vi "CANopen Read CAN Frame.vi"() -> ()   [LabVIEW 2016]
doc: "This example demonstrates how to read a raw CAN frame from CAN bus."
uses:
  <vilib>/userdefined/High Color/nirio_resource_hc.ctl
  <vilib>/Platform/TimedLoop/XDataNode/timing_clust.ctl
  <vilib>/Platform/TimedLoop/XDataNode/nitl_modes.ctl
  <vilib>/Platform/TimedLoop/XDataNode/wakeup.ctl
  <vilib>/FPGAPlugInAG/cRIO-9033/niLvFpga_Open_cRIO-9033.vi
  <vilib>/rvi/interface/common/dynamic/niFpgaDynamicAddResources.vi
  <vilib>/CANopenLib/CANOPEN.llb/CANopen Interface Create.vi
  <vilib>/CANopenLib/CANOPEN.llb/CANopen CAN Frame Read Create.vi
  <vilib>/CANopenLib/CANOPEN.llb/CANopen CAN Frame Read Start.vi
  <vilib>/CANopenLib/CANOPEN.llb/CANopen CAN Frame Read Close.vi
  <vilib>/CANopenLib/CANOPEN.llb/CANopen Interface Close.vi
  <vilib>/FPGAPlugInAG/Dynamic/niLvFpga_Close_Dynamic.vi
  <vilib>/rvi/interface/nirviOpenFPGA/nirviOpenFPGA.xnode
  FPGA Bitfiles/project_FPGATarget_MainFPGA_S9ZLErdeBuw.lvbitx
  FPGA/MainFPGA.vi
  <vilib>/Platform/TimedLoop/XDataNode/XDataNode.xnode
  <vilib>/rvi/interface/nirviCloseFPGA/nirviCloseFPGA.xnode
  <vilib>/Platform/TimedLoop/XDataNode/XDNodeRunTimeDep.lvlib
panel:
  in  "error in":errorcluster
  out "CAN message data":u8[](array[numeric])
  in  "period (ms)":i64=10
  out "COB-ID":u32 format="%.0x"
  out "RTR?":bool
  out "timestamp":timestamp
  out "New Data?":bool
  in  "stop":bool
  in  "buffer size (0)":u16=5
  in  "node-ID":u8=1 min=1 max=127 step=1
  in  "baud rate":u32(ring)=2 items=["1 Mbit/s"=0, "800 kbit/s"=1, "500 kbit/s"=2, "250 kbit/s"=3, "125 kbit/s"=4, "50 kbit/s"=6, "20 kbit/s"=7, "10 kbit/s"=8]
  in  "CANopen interface":u32(ring) items=["CANopen01", "CANopen02", "CANopen03", "CANopen04", "CANopen05", "CANopen06", "CANopen07", "CANopen08", "CANopen09", "CANopen10", "CANopen11", "CANopen12", "CANopen13", "CANopen14", "CANopen15", "CANopen16", "CANopen17", "CANopen18", "CANopen19", "CANopen20", "CANopen21", "CANopen22", "CANopen23", "CANopen24", "CANopen25", "CANopen26", "CANopen27", "CANopen28", "CANopen29", "CANopen30", "CANopen31", "CANopen32"]
  # "Overview: This example demonstrates how to read a raw CAN frame from CAN bus.  \nRequirements: Connect CANopen module with a slave device.\nInstructions:\n1. Specify the values of CANopen interface, baud rate of the CANopen interface, node-ID of the slave device and\n    buffer size (0) of the maximum number of CAN frames that the buffer saves.\n2. Run the VI.\n3. Click STOP to stop the VI."
  # "Create CANopen interface and raw CAN Frame object"
  # "Read CAN messages"
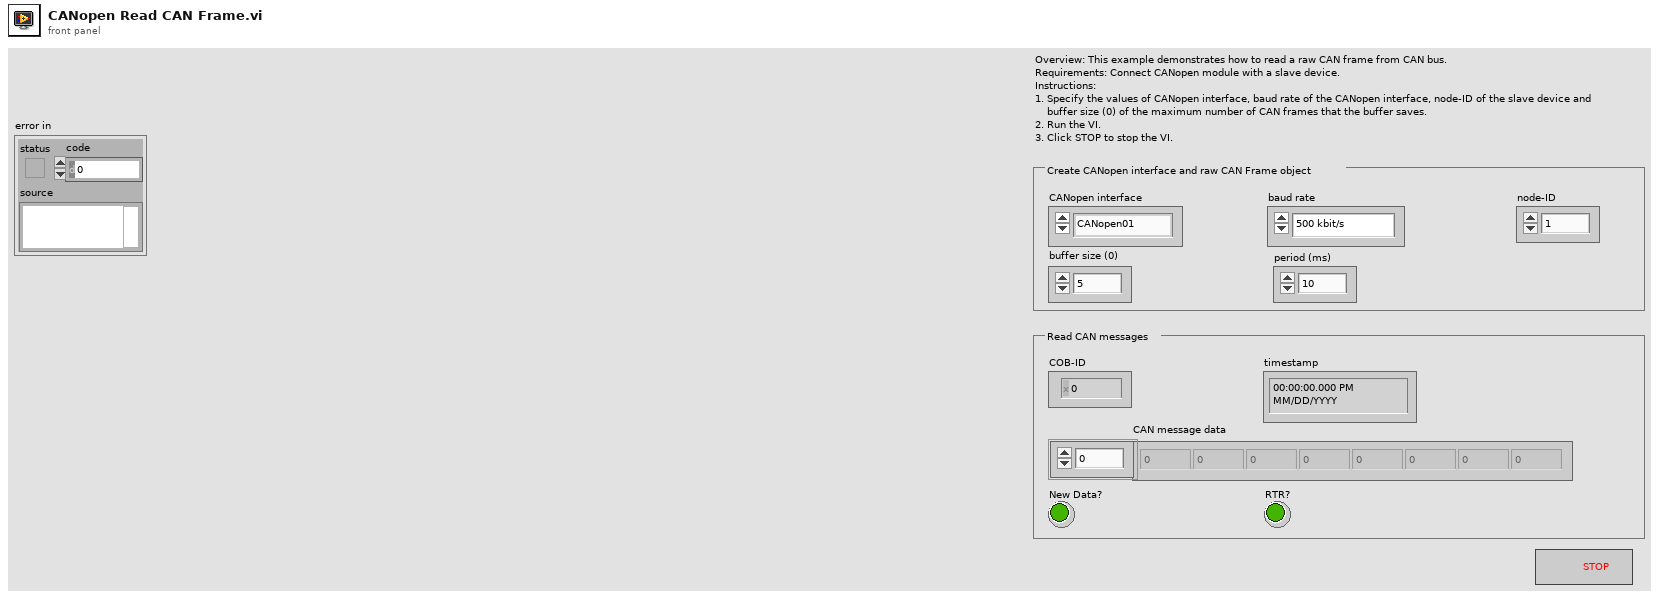
[diagram p1: front panel]
types:
  T1 = typedef "nirio_resource_hc.ctl" = tag
  T2 = typedef "XDNodeRunTimeDep.lvlib/timing_clust.ctl" = cluster{"Expected End [f-1]":u64, "Actual End [f-1]":u64, "Finished Late? [f-1]":bool, "Expected End [i-1]":u64, "Actual End [i-1]":u64, "Finished Late? [i-1]":bool, "Expected Start [i]":u64, "Actual Start [i]":u64, "Expected Start [f]":u64, "Actual Start [f]":u64, "Source Name":string, "Structure Name":string, "Period":i64, "Deadline":i64, "Offset":i64, "Start":i64, "Priority":i32, "Timeout":i32, "Mode":T3, "Wakeup Reason":T4, "Error":errorcluster, "Source Type":string, "Secondary Source Type":string, "Global End Time":u64, "Global Start Time":u64, "Frame Duration":u64, "Iteration Duration":u64, "Assigned CPU":i32, "I/O Scan Engine Mode":u32}
  T3 = typedef "XDNodeRunTimeDep.lvlib/nitl_modes.ctl" = enum32{"No Change", "Process missed periods, maintain original phase", "Discard missed periods, maintain original phase", "Process missed periods, ignore original phase", "Discard missed periods, ignore original phase"}
  T4 = typedef "XDNodeRunTimeDep.lvlib/wakeup.ctl" = enum32{"Normal", "Aborted", "Asynchronous wakeup", "Timing source error", "Timed loop error", "Timeout"}
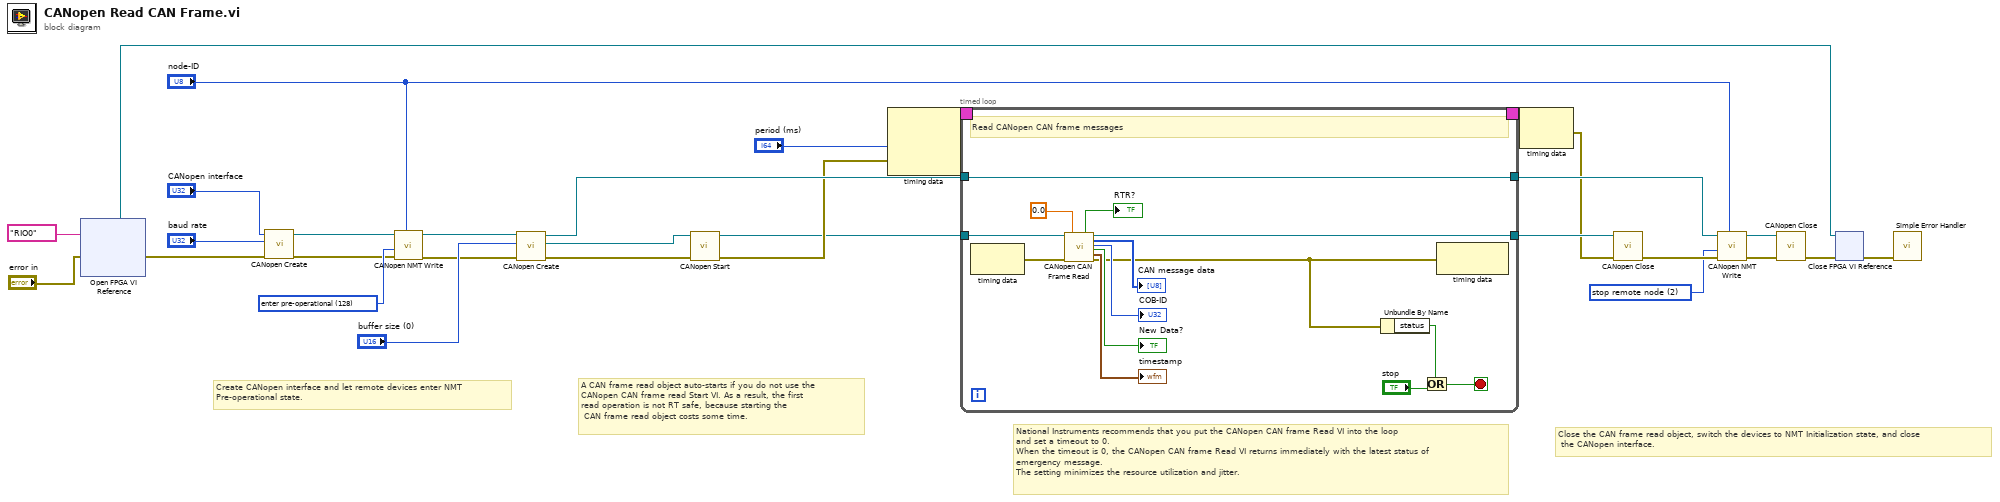
[diagram p0: block diagram]
diagram:
  w15 = u16 2 items=["start remote node"=1, "stop remote node"=2, "enter pre-operational"=128, "reset node"=129, "reset communication"=130] ("command")
  w26 = u16 128 items=["start remote node"=1, "stop remote node"=2, "enter pre-operational"=128, "reset node"=129, "reset communication"=130] ("command")
  # "A CAN frame read object auto-starts if you do not use the \nCANopen CAN frame read Start VI. As a result, the first \nread operation is not RT safe, because starting the\n CAN frame read object costs some time."
  # "Close the CAN frame read object, switch the devices to NMT Initialization state, and close\n the CANopen interface."
  # "Create CANopen interface and let remote devices enter NMT\nPre-operational state."
  # "National Instruments recommends that you put the CANopen CAN frame Read VI into the loop \nand set a timeout to 0.\nWhen the timeout is 0, the CANopen CAN frame Read VI returns immediately with the latest status of \nemergency message.\nThe setting minimizes the resource utilization and jitter."
  n1 = xnode ("Open FPGA VI Reference")("error in"="error in", "resource name"=T1 "RIO0") -> ("FPGA VI Reference Out"=w1:refnum<k20>, "error out"=w4:errorcluster)
  n2 = call-poly <vilib>:"CANopen Create.vi"("error in (no error)"=w4, "baud rate"="baud rate", "interface name"="CANopen interface") -> ("error out"=w25:errorcluster, "interface object out"=w24:refnum<k20>)  [unwired: 7 in]
  n3 = call <vilib>:"CANopen NMT Write.vi"("node-ID (0)"="node-ID", "error in (no error)"=w25, "command"=w26, "interface object in"=w24) -> ("error out"=w21:errorcluster, "interface object out"=w20:refnum<k20>)  [unwired: 6 in]
  n4 = call-poly <vilib>:"CANopen Create.vi"("error in (no error)"=w21, "buffer size (0)"="buffer size (0)", "interface object in"=w20) -> ("error out"=w12:errorcluster, "CAN frame read object out"=w11:refnum<k20>, "interface object out"=w19:refnum<k20>)  [unwired: 6 in]
  n5 = call-poly <vilib>:"CANopen Start.vi"("error in (no error)"=w12, "CAN frame read object in"=w11) -> ("error out"=w10:errorcluster, "CAN frame read object out"=w9:refnum<k20>)  [unwired: 8 in]
  n6 = node-c288("period (ms)", w10) -> (w30:T2)  [unwired: 1 in]
  n7 = timed-loop {
    timing: w30 -> [_]
    timing-out: [_] -> w29
    tunnel: [w44] -> w22
    tunnel: w19 -> [w36]
    tunnel: [w36] -> w13
    tunnel: w9 -> [w32]
    stop <- w38 stop-if-true
    # "Read CANopen CAN frame messages"
    n8 = node-c288() -> (w33:errorcluster)  [unwired: 1 in]
    n9 = call <vilib>:"CANopen CAN Frame Read.vi"("CAN frame read object in"=w32, "error in (no error)"=w33, "timeout (0s)"=0.0 ("timeout(0)")) -> ("RTR?"=→"RTR?":bool, "CAN frame read object out"=w44:refnum<k20>, "CAN message data"=→"CAN message data":u8[], "COB-ID"=→"COB-ID":u32, "new data?"=→"New Data?":bool, "timestamp"=→"timestamp":timestamp, "error out"=w31:errorcluster)  [unwired: 10 in]
    n10 = Unbundle By Name(w31) -> ("status"=w37:bool)
    n11 = Or(x=w37, y="stop") -> (x .or. y?=w38:bool)
    n12 = node-c288(w31) -> ()  [unwired: 1 out]
  }
  n13 = node-c288(w29) -> (w8:errorcluster)
  n14 = call-poly <vilib>:"CANopen Close.vi"("error in (no error)"=w8, "CAN frame read object in"=w22) -> ("error out"=w17:errorcluster)  [unwired: 9 in]
  n15 = call <vilib>:"CANopen NMT Write.vi"("node-ID (0)"="node-ID", "error in (no error)"=w17, "command"=w15, "interface object in"=w13) -> ("error out"=w16:errorcluster, "interface object out"=w18:refnum<k20>)  [unwired: 6 in]
  n16 = call-poly <vilib>:"CANopen Close.vi"("error in (no error)"=w16, "interface object in"=w18) -> ("error out"=w3:errorcluster)  [unwired: 9 in]
  n17 = xnode "Close FPGA VI Reference"("FPGA VI Reference In"=w1, "error in"=w3) -> ("error out"=w2:errorcluster)
  n18 = call <vilib>:"Simple Error Handler.vi"("error in (no error)"=w2) -> ()  [unwired: 4 in, 5 out]
